vi "S2DS_ReadScript.vi"(7 "Data save info (in)":T1={"File path"=path "", "Header"="", "File name"="", "False channel"=[], "Channel names"=[], "Buffer size"=0, "Format"="%.6f"}, 10 "All channel parameters":T2 {"Scan parameters"."Y data taking" items=["in both direction", "in up direction only", "in down direction only"]; "Scan parameters"."X data taking" items=["in both direction", "in up direction only", "in down direction only"]}, 11 "Status":refnum<vi>) -> (0 "Full Status":string, 1 "update instruction":i32[](array[numeric])=[0, 1, 2, 3, 4], 2 "All channel parameters (out)":T2 {"Scan parameters"."Y data taking" items=["in both direction", "in up direction only", "in down direction only"]; "Scan parameters"."X data taking" items=["in both direction", "in up direction only", "in down direction only"]}, 3 "Script complete?":bool, 5 "Data save info (out)":T1={"File path"=path "", "Header"="", "File name"="", "False channel"=[], "Channel names"=[], "Buffer size"=0, "Format"="%.6f"})   [LabVIEW 2025]
uses:
  TYPE DEFS/S2DS_All Channel Parameters.ctl
  TYPE DEFS/S2DS_WC info.ctl
  TYPE DEFS/S2DS_Single WC info.ctl
  TYPE DEFS/S2DS_RC info.ctl
  TYPE DEFS/S2DS_Single RC info.ctl
  TYPE DEFS/S2DS_DAC info new.ctl
  TYPE DEFS/S2DS_Single DC info.ctl
  TYPE DEFS/S2DS_Array Inst Info.ctl
  TYPE DEFS/S2DS_Sweep Info.ctl
  TYPE DEFS/S2DS_Data saving info.ctl
  <vilib>/Utility/error.llb/Trim Whitespace One-Sided.vi
  <vilib>/Utility/config.llb/Read Key (Path).vi
  <vilib>/Utility/config.llb/Read Key (I32).vi
  <vilib>/Utility/config.llb/Write Key (Path).vi
  <vilib>/Utility/config.llb/Read Key (String).vi
  <vilib>/Utility/config.llb/Write Key (I32).vi
  <vilib>/Utility/config.llb/NI_LVConfig.lvlib
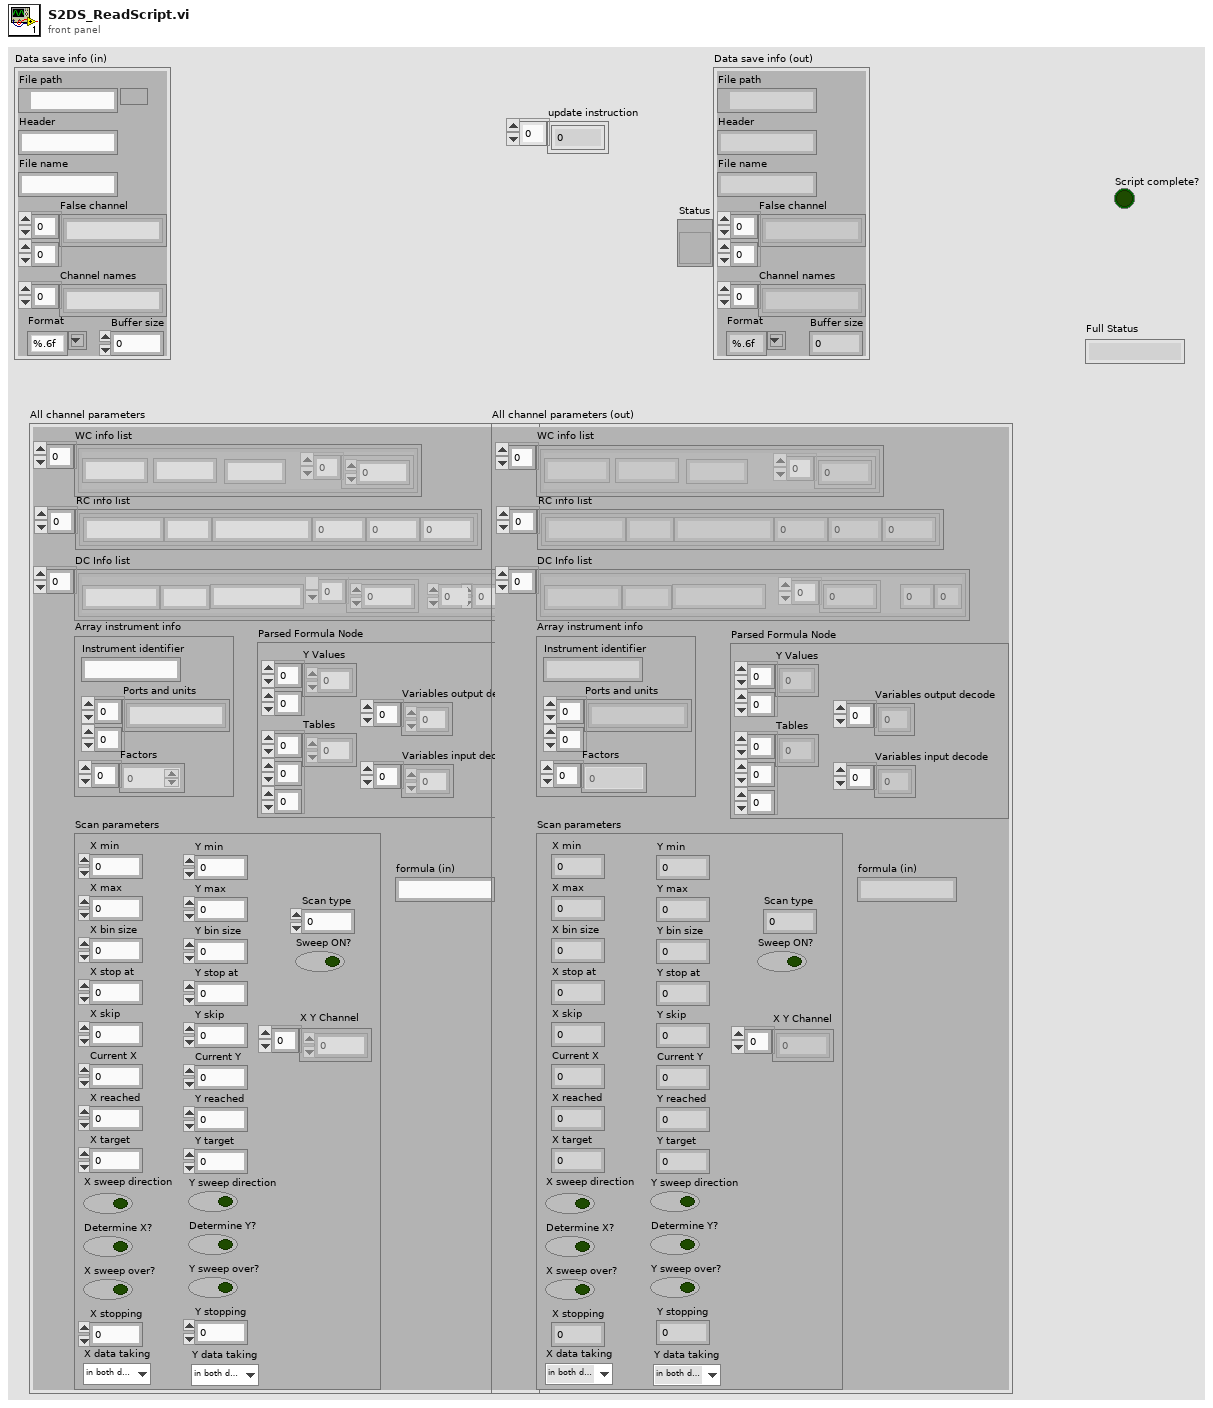
[diagram p1: front panel]
types:
  T1 = typedef "S2DS_Data saving info.ctl" = cluster{"File path":path, "Header":string, "File name":string, "False channel":string[][], "Channel names":string[], "Buffer size":i32, "Format":string}
  T2 = typedef "S2DS_All Channel Parameters.ctl" = cluster{"WC info list":T3, "RC info list":T5, "DC Info list":T7, "Array instrument info":T9, "Scan parameters":T10, "Parsed Formula Node":cluster{"Y Values":dbl[][], "Tables":i32[][][], "Variables input decode":i32[], "Variables output decode":i32[]}, "formula (in)":string}
  T3 = typedef "S2DS_WC info.ctl" = T4[]
  T4 = typedef "S2DS_Single WC info.ctl" = cluster{"Instrument identifier":string, "Write channel parameters":dbl[], "Name":string, "Unit":string}
  T5 = typedef "S2DS_RC info.ctl" = T6[]
  T6 = typedef "S2DS_Single RC info.ctl" = cluster{"Instrument identifier":string, "Factor":dbl, "Averaging":i32, "Wait (ms)":i32, "Unit":string, "Name":string}
  T7 = typedef "S2DS_DAC info new.ctl" = T8[]
  T8 = typedef "S2DS_Single DC info.ctl" = cluster{"Operation identifier":string, "DC parameters":dbl[], "U":i32, "V":i32, "Name":string, "Unit":string}
  T9 = typedef "S2DS_Array Inst Info.ctl" = cluster{"Instrument identifier":string, "Ports and units":string[][], "Factors":dbl[]}
  T10 = typedef "S2DS_Sweep Info.ctl" = cluster{"X min":ext, "X max":dbl, "Y min":dbl, "Y max":dbl, "X bin size":dbl, "Y bin size":dbl, "X stop at":dbl, "Y stop at":dbl, "X skip":u64, "Y skip":u64, "Current X":dbl, "Current Y":dbl, "X reached":i32, "Y reached":i32, "X target":dbl, "Y target":dbl, "Sweep ON?":bool, "X sweep direction":bool, "Y sweep direction":bool, "Determine X?":bool, "Determine Y?":bool, "X sweep over?":bool, "Y sweep over?":bool, "Scan type":i32, "X stopping":i32, "Y stopping":i32, "X Y Channel":u16[], "X data taking":u16, "Y data taking":u16}
  T11 = typedef "NI_LVConfig.lvlib/Config Data RefNum.ctl" = refnum<k1>
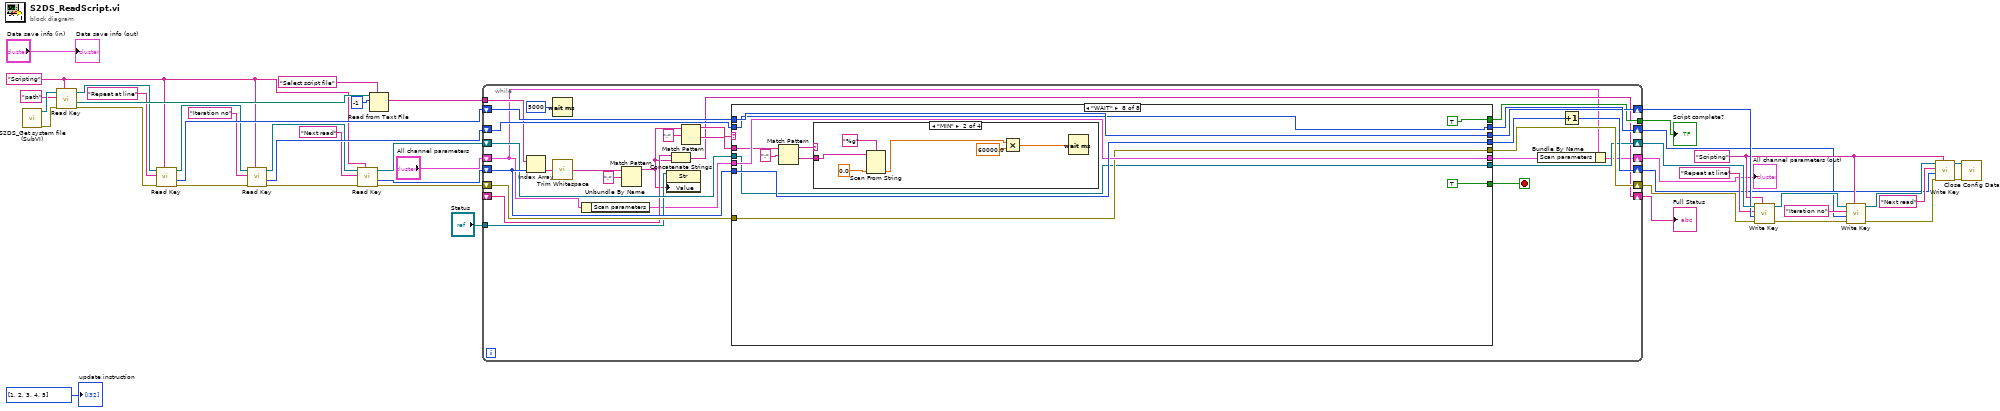
[diagram p0: block diagram]
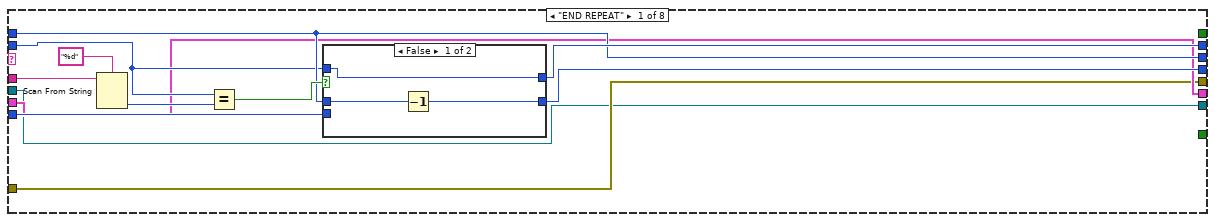
[diagram p2: hidden frame]
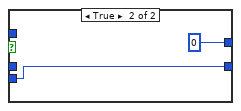
[diagram p3: hidden frame]
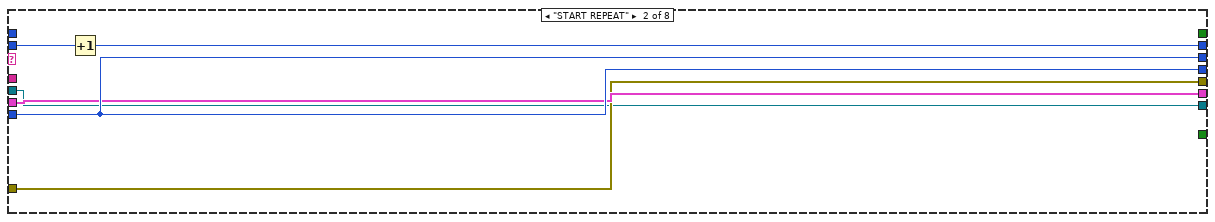
[diagram p4: hidden frame]
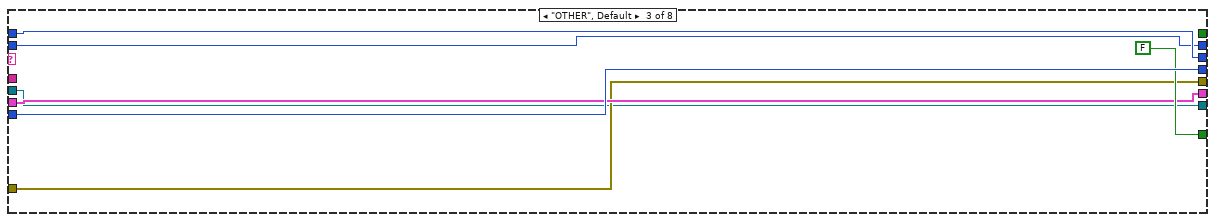
[diagram p5: hidden frame]
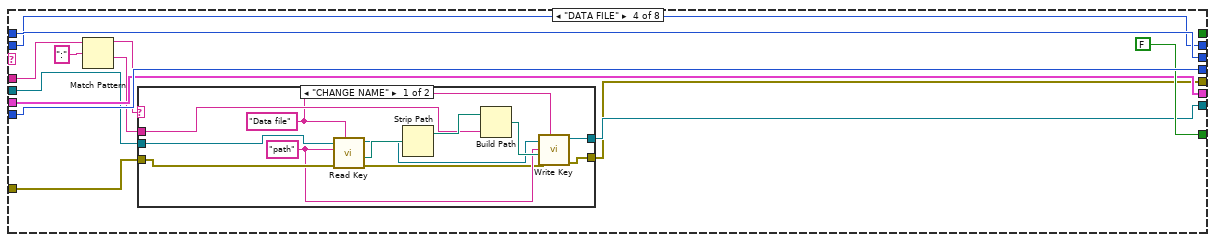
[diagram p6: hidden frame]
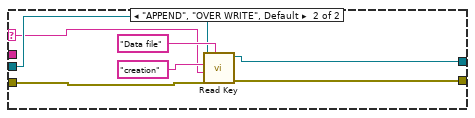
[diagram p7: hidden frame]
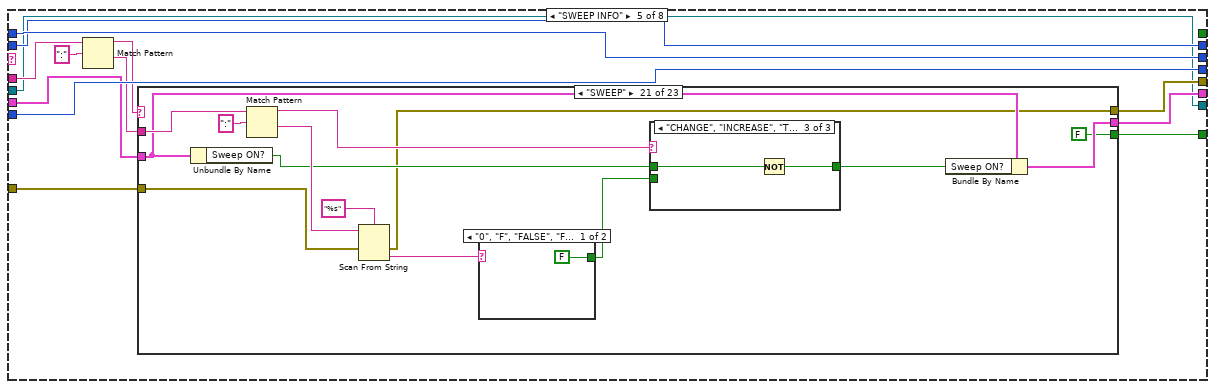
[diagram p8: hidden frame]
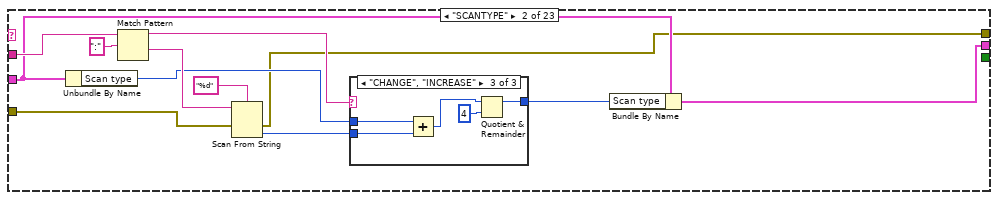
[diagram p10: hidden frame]
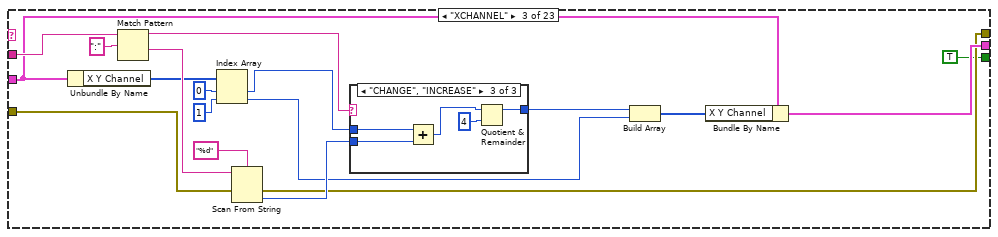
[diagram p13: hidden frame]
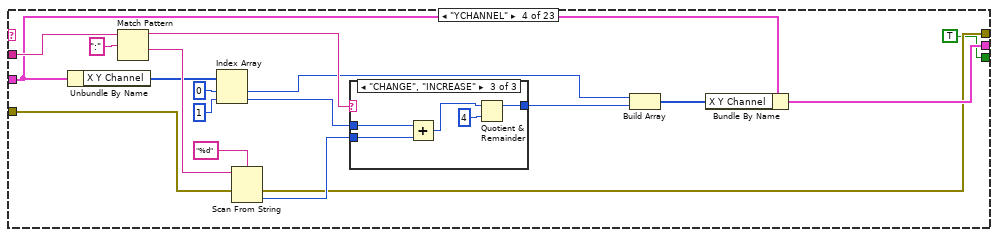
[diagram p16: hidden frame]
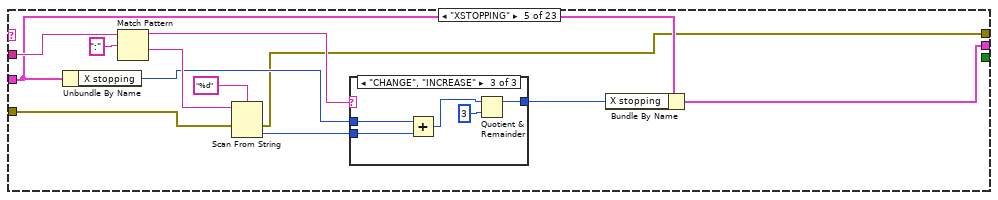
[diagram p19: hidden frame]
diagram:
  w12 = "Scripting" ("section")
  w27 = "Scripting" ("section")
  n1 = call "S2DS_Get system file (SubVI).vi"() -> ("error out"=w39:errorcluster, "Refnum out"=w40:T11)  [unwired: 10 in]
  n2 = call-poly <vilib>:"Read Key.vi"("section"=w27, "error in (no error)"=w39, "key"="path", "refnum"=w40) -> ("error out"=w35:errorcluster, "value"=w37:path, "refnum out"=w36:T11)  [unwired: 4 in, 1 out]
  n3 = call-poly <vilib>:"Read Key.vi"("section"=w27, "error in (no error)"=w35, "key"="Repeat at line", "refnum"=w36) -> ("error out"=w30:errorcluster, "value"=w33:i32, "refnum out"=w32:T11)  [unwired: 4 in, 1 out]
  n4 = call-poly <vilib>:"Read Key.vi"("section"=w27, "error in (no error)"=w30, "key"="Iteration no", "refnum"=w32) -> ("error out"=w25:errorcluster, "value"=w29:i32, "refnum out"=w28:T11)  [unwired: 4 in, 1 out]
  n5 = call-poly <vilib>:"Read Key.vi"("section"=w27, "error in (no error)"=w25, "key"="Next read", "refnum"=w28) -> ("error out"=w23:errorcluster, "value"=w24:i32, "refnum out"=w22:T11)  [unwired: 4 in, 1 out]
  n6 = Read from Text File(prompt (Open existing file)="Select script file" ("prompt"), file (use dialog)=w37, count=-1) -> (text=w42:string[])  [unwired: 1 in, 3 out]
  n7 = while {
    tunnel: w42 -> [w66]
    shift-right: [w69] -> w5
    shift-left: w29 -> [w70]
    shift-right: [w62] -> w6
    shift-left: w24 -> [w65]
    shift-right: [w68] -> w19
    shift-left: w33 -> [w67]
    tunnel: [w57] -> w41
    shift-right: [w45] -> w2
    shift-left: "All channel parameters" -> [w47]
    shift-right: [w55] -> w20
    shift-left: w23 -> [w56]
    shift-right: [w53] -> w21
    shift-left: w22 -> [w54]
    shift-right: [w51] -> w8
    shift-left: _ -> [w52]
    tunnel: "Status" -> [w50]
    stop <- w61 stop-if-true
    n8 = Index Array(array=w66, index=w65) -> (element=w64:string)
    n9 = Wait (ms)(milliseconds to wait=u32 5000) -> ()  [unwired: 1 out]
    n10 = call <vilib>:"Trim Whitespace.vi"("string"=w64) -> ("trimmed string"=w59:string)  [unwired: 1 in]
    n11 = Unbundle By Name(w47) -> ("Scan parameters"=w48:T10)
    n12 = Match Pattern(string=w59, regular expression=";") -> (before substring=w49:string)  [unwired: 1 in, 3 out]
    n13 = property on="Property Node" class="Str"(reference=w50, "Value"=w49) -> ()  [unwired: 1 in, 2 out]
    n14 = Concatenate Strings(w52, w49) -> (w51:string)
    n15 = Match Pattern(string=w49, regular expression=":") -> (before substring=w60:string, after substring=w71:string)  [unwired: 1 in, 2 out]
    n16 = case shown="\"WAIT\"" w60 {
      tunnel: w71 -> [w83 _ _ w110 w145 _ _ w571]
      tunnel: w70 -> [w77 w96 w101 w114 w146 w558 w566 w578]
      tunnel: [w79 w95 w101 w114 w146 w558 w566 w578] -> w69
      tunnel: [w78 w94 w102 w115 w147 w559 w567 w579] -> w68
      tunnel: w65 -> [w85 w94 w103 w116 w148 w560 w568 w580]
      tunnel: w67 -> [w78 _ w102 w115 w147 w559 w567 w579]
      tunnel: [w84 w94 w103 w116 w148 w560 w568 w580] -> w63
      tunnel: [_ _ FALSE FALSE w137 TRUE TRUE TRUE] -> w61
      tunnel: [_ _ _ _ _ _ TRUE TRUE] -> w57
      tunnel: w48 -> [w76 w93 w99 w112 w142 w556 w563 w575]
      tunnel: [w76 w93 w99 w112 w141 w556 w563 w575] -> w46
      tunnel: w56 -> [w75 w92 w98 w105 w140 w555 w562 w574]
      tunnel: [w75 w92 w98 w104 w139 w555 w562 w574] -> w55
      tunnel: w54 -> [w74 w91 w97 w108 w136 w554 w561 w573]
      tunnel: [w74 w91 w97 w106 w136 w554 w561 w573] -> w53
      frame "END REPEAT" {
        n17 = Scan From String(format string="%d", input string=w83) -> (output 1=w81:i32)  [unwired: 3 in, 3 out]
        n18 = Equal?(x=w77, y=w81) -> (x = y?=w80:bool)
        n19 = case shown="False" w80 {
          tunnel: w85 -> [_ w89]
          tunnel: [w86 w89] -> w84
          tunnel: w78 -> [w87 _]
          tunnel: [w88 0] -> w79
          tunnel: w77 -> [w88 _]
          frame False {
            n20 = Decrement(x=w87) -> (x-1=w86:i32)
          }
          frame True {
          }
        }
      }
      frame "START REPEAT" {
        n21 = Increment(x=w96) -> (x+1=w95:i32)
      }
      frame "OTHER", Default {
      }
      frame "DATA FILE" {
        n22 = Match Pattern(string=w110, regular expression=":") -> (before substring=w109:string, after substring=w107:string)  [unwired: 1 in, 2 out]
        n23 = case shown="\"CHANGE NAME\"" w109 {
          selector: w109 -> [_ w131]
          tunnel: w107 -> [w124 _]
          tunnel: w108 -> [w128 w133]
          tunnel: w105 -> [w127 w132]
          tunnel: [w118 w130] -> w106
          tunnel: [w117 w129] -> w104
          frame "CHANGE NAME" {
            w121 = "path" ("key")
            w122 = "Data file" ("section")
            n24 = call-poly <vilib>:"Read Key.vi"("section"=w122, "error in (no error)"=w127, "key"=w121, "refnum"=w128) -> ("error out"=w119:errorcluster, "value"=w126:path, "refnum out"=w120:T11)  [unwired: 4 in, 1 out]
            n25 = Strip Path(path=w126) -> (stripped path=w125:path)  [unwired: 1 out]
            n26 = Build Path(base path=w125, name or relative path=w124) -> (appended path=w123:path)
            n27 = call-poly <vilib>:"Write Key.vi"("section"=w122, "error in (no error)"=w119, "value"=w123, "key"=w121, "refnum"=w120) -> ("error out"=w117:errorcluster, "refnum out"=w118:T11)  [unwired: 4 in, 1 out]
          }
          frame "APPEND", "OVER WRITE", Default {
            n28 = call-poly <vilib>:"Read Key.vi"("section"="Data file", "error in (no error)"=w132, "default value"=w131, "key"="creation", "refnum"=w133) -> ("error out"=w129:errorcluster, "refnum out"=w130:T11)  [unwired: 3 in, 2 out]
          }
        }
      }
      frame "SWEEP INFO" {
        n29 = Match Pattern(string=w145, regular expression=":") -> (before substring=w143:string, after substring=w138:string)  [unwired: 1 in, 2 out]
        n30 = case shown="\"SWEEP\"" w143 {
          tunnel: w138 -> [_ w162 w187 w212 w231 w250 w269 w286 w303 w320 w337 w354 w371 w388 w405 w422 w439 w456 w473 w490 w509 w528 w547]
          tunnel: w142 -> [w150 w157 w182 w207 w226 w245 w264 w281 w298 w315 w332 w349 w366 w383 w400 w417 w434 w451 w468 w485 w504 w523 w542]
          tunnel: [w150 w156 w181 w206 w225 w244 w263 w280 w297 w314 w331 w348 w365 w382 w399 w416 w433 w450 w467 w484 w503 w522 w541] -> w141
          tunnel: w140 -> [w149 w152 w179 w204 w221 w240 w259 w276 w293 w310 w327 w344 w361 w378 w395 w412 w429 w446 w463 w480 w500 w519 w538]
          tunnel: [w149 w151 w178 w203 w220 w239 w258 w275 w292 w309 w326 w343 w360 w377 w394 w411 w428 w445 w462 w479 w499 w518 w537] -> w139
          tunnel: [_ _ TRUE TRUE _ _ _ _ _ _ _ _ _ _ _ _ _ _ _ _ FALSE _ _] -> w137
          frame "False", Default {
          }
          frame "SCANTYPE" {
            n31 = Unbundle By Name(w157) -> ("Scan type"=w154:i32)
            n32 = Match Pattern(string=w162, regular expression=":") -> (before substring=w161:string, after substring=w159:string)  [unwired: 1 in, 2 out]
            n33 = Scan From String(format string="%d", input string=w159, error in=w152) -> (error out=w151:errorcluster, output 1=w153:i32)  [unwired: 2 in, 2 out]
            n34 = case shown="\"CHANGE\", \"INCREASE\"" w161 {
              tunnel: [w163 w164 w165] -> w155
              tunnel: w154 -> [w163 _ w168]
              tunnel: w153 -> [_ w164 w169]
              frame "False", Default {
              }
              frame "SET" {
              }
              frame "CHANGE", "INCREASE" {
                n35 = Add(x=w168, y=w169) -> (x+y=w167:i32)
                n36 = Quotient & Remainder(x=w167, y=4) -> (x-y*floor(x/y)=w165:i32)  [unwired: 1 out]
              }
            }
            n37 = Bundle By Name(cluster=w157, "Scan type"=w155) -> (w156:T10)
          }
          frame "XCHANNEL" {
            n38 = Unbundle By Name(w182) -> ("X Y Channel"=w177:u16[])
            n39 = Match Pattern(string=w187, regular expression=":") -> (before substring=w186:string, after substring=w184:string)  [unwired: 1 in, 2 out]
            n40 = Index Array(array=w177, index #1=0 ("index"), index #2=1 ("index")) -> (element #1=w174:u16, element #2=w172:u16)
            n41 = Scan From String(format string="%d", input string=w184, error in=w179) -> (error out=w178:errorcluster, output 1=w180:i32)  [unwired: 2 in, 2 out]
            n42 = case shown="\"CHANGE\", \"INCREASE\"" w186 {
              tunnel: [w188 w189 w190] -> w173
              tunnel: w174 -> [w188 _ w193]
              tunnel: w180 -> [_ w189 w194]
              frame "False", Default {
              }
              frame "SET" {
              }
              frame "CHANGE", "INCREASE" {
                n43 = Add(x=w193, y=w194) -> (x+y=w192:i32)
                n44 = Quotient & Remainder(x=w192, y=4) -> (x-y*floor(x/y)=w190:i32)  [unwired: 1 out]
              }
            }
            n45 = Build Array(w173, w172) -> (w171:i32[])
            n46 = Bundle By Name(cluster=w182, "X Y Channel"=w171) -> (w181:T10)
          }
          frame "YCHANNEL" {
            n47 = Unbundle By Name(w207) -> ("X Y Channel"=w202:u16[])
            n48 = Match Pattern(string=w212, regular expression=":") -> (before substring=w211:string, after substring=w209:string)  [unwired: 1 in, 2 out]
            n49 = Index Array(array=w202, index #1=0 ("index"), index #2=1 ("index")) -> (element #1=w196:u16, element #2=w198:u16)
            n50 = Scan From String(format string="%d", input string=w209, error in=w204) -> (error out=w203:errorcluster, output 1=w205:i32)  [unwired: 2 in, 2 out]
            n51 = case shown="\"CHANGE\", \"INCREASE\"" w211 {
              tunnel: [w213 w214 w215] -> w197
              tunnel: w198 -> [w213 _ w218]
              tunnel: w205 -> [_ w214 w219]
              frame "False", Default {
              }
              frame "SET" {
              }
              frame "CHANGE", "INCREASE" {
                n52 = Add(x=w218, y=w219) -> (x+y=w217:i32)
                n53 = Quotient & Remainder(x=w217, y=4) -> (x-y*floor(x/y)=w215:i32)  [unwired: 1 out]
              }
            }
            n54 = Build Array(w196, w197) -> (w199:i32[])
            n55 = Bundle By Name(cluster=w207, "X Y Channel"=w199) -> (w206:T10)
          }
          frame "XSTOPPING" {
            n56 = Unbundle By Name(w226) -> ("X stopping"=w223:i32)
            n57 = Match Pattern(string=w231, regular expression=":") -> (before substring=w230:string, after substring=w228:string)  [unwired: 1 in, 2 out]
            n58 = Scan From String(format string="%d", input string=w228, error in=w221) -> (error out=w220:errorcluster, output 1=w222:i32)  [unwired: 2 in, 2 out]
            n59 = case shown="\"CHANGE\", \"INCREASE\"" w230 {
              tunnel: [w232 w233 w234] -> w224
              tunnel: w223 -> [w232 _ w237]
              tunnel: w222 -> [_ w233 w238]
              frame "False", Default {
              }
              frame "SET" {
              }
              frame "CHANGE", "INCREASE" {
                n60 = Add(x=w237, y=w238) -> (x+y=w236:i32)
                n61 = Quotient & Remainder(x=w236, y=3) -> (x-y*floor(x/y)=w234:i32)  [unwired: 1 out]
              }
            }
            n62 = Bundle By Name(cluster=w226, "X stopping"=w224) -> (w225:T10)
          }
          frame "YSTOPPING" {
            n63 = Unbundle By Name(w245) -> ("Y stopping"=w242:i32)
            n64 = Match Pattern(string=w250, regular expression=":") -> (before substring=w249:string, after substring=w247:string)  [unwired: 1 in, 2 out]
            n65 = Scan From String(format string="%d", input string=w247, error in=w240) -> (error out=w239:errorcluster, output 1=w241:i32)  [unwired: 2 in, 2 out]
            n66 = case shown="\"CHANGE\", \"INCREASE\"" w249 {
              tunnel: [w251 w252 w253] -> w243
              tunnel: w242 -> [w251 _ w256]
              tunnel: w241 -> [_ w252 w257]
              frame "False", Default {
              }
              frame "SET" {
              }
              frame "CHANGE", "INCREASE" {
                n67 = Add(x=w256, y=w257) -> (x+y=w255:i32)
                n68 = Quotient & Remainder(x=w255, y=3) -> (x-y*floor(x/y)=w253:i32)  [unwired: 1 out]
              }
            }
            n69 = Bundle By Name(cluster=w245, "Y stopping"=w243) -> (w244:T10)
          }
          frame "XMIN" {
            n70 = Unbundle By Name(w264) -> ("X min"=w261:ext)
            n71 = Match Pattern(string=w269, regular expression=":") -> (before substring=w268:string, after substring=w266:string)  [unwired: 1 in, 2 out]
            n72 = Scan From String(format string="%g", input string=w266, error in=w259) -> (error out=w258:errorcluster, output 1=w260:dbl)  [unwired: 2 in, 2 out]
            n73 = case shown="\"CHANGE\", \"INCREASE\"" w268 {
              tunnel: [w270 w271 w272] -> w262
              tunnel: w261 -> [w270 _ w273]
              tunnel: w260 -> [_ w271 w274]
              frame "False", Default {
              }
              frame "SET" {
              }
              frame "CHANGE", "INCREASE" {
                n74 = Add(x=w273, y=w274) -> (x+y=w272:ext)
              }
            }
            n75 = Bundle By Name(cluster=w264, "X min"=w262) -> (w263:T10)
          }
          frame "XMAX" {
            n76 = Unbundle By Name(w281) -> ("X max"=w278:dbl)
            n77 = Match Pattern(string=w286, regular expression=":") -> (before substring=w285:string, after substring=w283:string)  [unwired: 1 in, 2 out]
            n78 = Scan From String(format string="%g", input string=w283, error in=w276) -> (error out=w275:errorcluster, output 1=w277:dbl)  [unwired: 2 in, 2 out]
            n79 = case shown="\"CHANGE\", \"INCREASE\"" w285 {
              tunnel: [w287 w288 w289] -> w279
              tunnel: w278 -> [w287 _ w290]
              tunnel: w277 -> [_ w288 w291]
              frame "False", Default {
              }
              frame "SET" {
              }
              frame "CHANGE", "INCREASE" {
                n80 = Add(x=w290, y=w291) -> (x+y=w289:dbl)
              }
            }
            n81 = Bundle By Name(cluster=w281, "X max"=w279) -> (w280:T10)
          }
          frame "YMIN" {
            n82 = Unbundle By Name(w298) -> ("Y min"=w295:dbl)
            n83 = Match Pattern(string=w303, regular expression=":") -> (before substring=w302:string, after substring=w300:string)  [unwired: 1 in, 2 out]
            n84 = Scan From String(format string="%g", input string=w300, error in=w293) -> (error out=w292:errorcluster, output 1=w294:dbl)  [unwired: 2 in, 2 out]
            n85 = case shown="\"CHANGE\", \"INCREASE\"" w302 {
              tunnel: [w304 w305 w306] -> w296
              tunnel: w295 -> [w304 _ w307]
              tunnel: w294 -> [_ w305 w308]
              frame "False", Default {
              }
              frame "SET" {
              }
              frame "CHANGE", "INCREASE" {
                n86 = Add(x=w307, y=w308) -> (x+y=w306:dbl)
              }
            }
            n87 = Bundle By Name(cluster=w298, "Y min"=w296) -> (w297:T10)
          }
          frame "YMAX" {
            n88 = Unbundle By Name(w315) -> ("Y max"=w312:dbl)
            n89 = Match Pattern(string=w320, regular expression=":") -> (before substring=w319:string, after substring=w317:string)  [unwired: 1 in, 2 out]
            n90 = Scan From String(format string="%g", input string=w317, error in=w310) -> (error out=w309:errorcluster, output 1=w311:dbl)  [unwired: 2 in, 2 out]
            n91 = case shown="\"CHANGE\", \"INCREASE\"" w319 {
              tunnel: [w321 w322 w323] -> w313
              tunnel: w312 -> [w321 _ w324]
              tunnel: w311 -> [_ w322 w325]
              frame "False", Default {
              }
              frame "SET" {
              }
              frame "CHANGE", "INCREASE" {
                n92 = Add(x=w324, y=w325) -> (x+y=w323:dbl)
              }
            }
            n93 = Bundle By Name(cluster=w315, "Y max"=w313) -> (w314:T10)
          }
          frame "XBIN" {
            n94 = Unbundle By Name(w332) -> ("X bin size"=w329:dbl)
            n95 = Match Pattern(string=w337, regular expression=":") -> (before substring=w336:string, after substring=w334:string)  [unwired: 1 in, 2 out]
            n96 = Scan From String(format string="%g", input string=w334, error in=w327) -> (error out=w326:errorcluster, output 1=w328:dbl)  [unwired: 2 in, 2 out]
            n97 = case shown="\"CHANGE\", \"INCREASE\"" w336 {
              tunnel: [w338 w339 w340] -> w330
              tunnel: w329 -> [w338 _ w341]
              tunnel: w328 -> [_ w339 w342]
              frame "False", Default {
              }
              frame "SET" {
              }
              frame "CHANGE", "INCREASE" {
                n98 = Add(x=w341, y=w342) -> (x+y=w340:dbl)
              }
            }
            n99 = Bundle By Name(cluster=w332, "X bin size"=w330) -> (w331:T10)
          }
          frame "YBIN" {
            n100 = Unbundle By Name(w349) -> ("Y bin size"=w346:dbl)
            n101 = Match Pattern(string=w354, regular expression=":") -> (before substring=w353:string, after substring=w351:string)  [unwired: 1 in, 2 out]
            n102 = Scan From String(format string="%g", input string=w351, error in=w344) -> (error out=w343:errorcluster, output 1=w345:dbl)  [unwired: 2 in, 2 out]
            n103 = case shown="\"CHANGE\", \"INCREASE\"" w353 {
              tunnel: [w355 w356 w357] -> w347
              tunnel: w346 -> [w355 _ w358]
              tunnel: w345 -> [_ w356 w359]
              frame "False", Default {
              }
              frame "SET" {
              }
              frame "CHANGE", "INCREASE" {
                n104 = Add(x=w358, y=w359) -> (x+y=w357:dbl)
              }
            }
            n105 = Bundle By Name(cluster=w349, "Y bin size"=w347) -> (w348:T10)
          }
          frame "XSTOPPAGE" {
            n106 = Unbundle By Name(w366) -> ("X stop at"=w363:dbl)
            n107 = Match Pattern(string=w371, regular expression=":") -> (before substring=w370:string, after substring=w368:string)  [unwired: 1 in, 2 out]
            n108 = Scan From String(format string="%g", input string=w368, error in=w361) -> (error out=w360:errorcluster, output 1=w362:dbl)  [unwired: 2 in, 2 out]
            n109 = case shown="\"CHANGE\", \"INCREASE\"" w370 {
              tunnel: [w372 w373 w374] -> w364
              tunnel: w363 -> [w372 _ w375]
              tunnel: w362 -> [_ w373 w376]
              frame "False", Default {
              }
              frame "SET" {
              }
              frame "CHANGE", "INCREASE" {
                n110 = Add(x=w375, y=w376) -> (x+y=w374:dbl)
              }
            }
            n111 = Bundle By Name(cluster=w366, "X stop at"=w364) -> (w365:T10)
          }
          frame "YSTOPPAGE" {
            n112 = Unbundle By Name(w383) -> ("Y stop at"=w380:dbl)
            n113 = Match Pattern(string=w388, regular expression=":") -> (before substring=w387:string, after substring=w385:string)  [unwired: 1 in, 2 out]
            n114 = Scan From String(format string="%g", input string=w385, error in=w378) -> (error out=w377:errorcluster, output 1=w379:dbl)  [unwired: 2 in, 2 out]
            n115 = case shown="\"CHANGE\", \"INCREASE\"" w387 {
              tunnel: [w389 w390 w391] -> w381
              tunnel: w380 -> [w389 _ w392]
              tunnel: w379 -> [_ w390 w393]
              frame "False", Default {
              }
              frame "SET" {
              }
              frame "CHANGE", "INCREASE" {
                n116 = Add(x=w392, y=w393) -> (x+y=w391:dbl)
              }
            }
            n117 = Bundle By Name(cluster=w383, "Y stop at"=w381) -> (w382:T10)
          }
          frame "XSKIP" {
            n118 = Unbundle By Name(w400) -> ("X skip"=w397:u64)
            n119 = Match Pattern(string=w405, regular expression=":") -> (before substring=w404:string, after substring=w402:string)  [unwired: 1 in, 2 out]
            n120 = Scan From String(format string="%g", input string=w402, error in=w395) -> (error out=w394:errorcluster, output 1=w396:dbl)  [unwired: 2 in, 2 out]
            n121 = case shown="\"CHANGE\", \"INCREASE\"" w404 {
              tunnel: [w406 w407 w408] -> w398
              tunnel: w397 -> [w406 _ w409]
              tunnel: w396 -> [_ w407 w410]
              frame "False", Default {
              }
              frame "SET" {
              }
              frame "CHANGE", "INCREASE" {
                n122 = Add(x=w409, y=w410) -> (x+y=w408:dbl)
              }
            }
            n123 = Bundle By Name(cluster=w400, "X skip"=w398) -> (w399:T10)
          }
          frame "YSKIP" {
            n124 = Unbundle By Name(w417) -> ("Y skip"=w414:u64)
            n125 = Match Pattern(string=w422, regular expression=":") -> (before substring=w421:string, after substring=w419:string)  [unwired: 1 in, 2 out]
            n126 = Scan From String(format string="%g", input string=w419, error in=w412) -> (error out=w411:errorcluster, output 1=w413:dbl)  [unwired: 2 in, 2 out]
            n127 = case shown="\"CHANGE\", \"INCREASE\"" w421 {
              tunnel: [w423 w424 w425] -> w415
              tunnel: w414 -> [w423 _ w426]
              tunnel: w413 -> [_ w424 w427]
              frame "False", Default {
              }
              frame "SET" {
              }
              frame "CHANGE", "INCREASE" {
                n128 = Add(x=w426, y=w427) -> (x+y=w425:dbl)
              }
            }
            n129 = Bundle By Name(cluster=w417, "Y skip"=w415) -> (w416:T10)
          }
          frame "XPRESENT" {
            n130 = Unbundle By Name(w434) -> ("Current X"=w431:dbl)
            n131 = Match Pattern(string=w439, regular expression=":") -> (before substring=w438:string, after substring=w436:string)  [unwired: 1 in, 2 out]
            n132 = Scan From String(format string="%g", input string=w436, error in=w429) -> (error out=w428:errorcluster, output 1=w430:dbl)  [unwired: 2 in, 2 out]
            n133 = case shown="\"CHANGE\", \"INCREASE\"" w438 {
              tunnel: [w440 w441 w442] -> w432
              tunnel: w431 -> [w440 _ w443]
              tunnel: w430 -> [_ w441 w444]
              frame "False", Default {
              }
              frame "SET" {
              }
              frame "CHANGE", "INCREASE" {
                n134 = Add(x=w443, y=w444) -> (x+y=w442:dbl)
              }
            }
            n135 = Bundle By Name(cluster=w434, "Current X"=w432) -> (w433:T10)
          }
          frame "YPRESENT" {
            n136 = Unbundle By Name(w451) -> ("Current Y"=w448:dbl)
            n137 = Match Pattern(string=w456, regular expression=":") -> (before substring=w455:string, after substring=w453:string)  [unwired: 1 in, 2 out]
            n138 = Scan From String(format string="%g", input string=w453, error in=w446) -> (error out=w445:errorcluster, output 1=w447:dbl)  [unwired: 2 in, 2 out]
            n139 = case shown="\"CHANGE\", \"INCREASE\"" w455 {
              tunnel: [w457 w458 w459] -> w449
              tunnel: w448 -> [w457 _ w460]
              tunnel: w447 -> [_ w458 w461]
              frame "False", Default {
              }
              frame "SET" {
              }
              frame "CHANGE", "INCREASE" {
                n140 = Add(x=w460, y=w461) -> (x+y=w459:dbl)
              }
            }
            n141 = Bundle By Name(cluster=w451, "Current Y"=w449) -> (w450:T10)
          }
          frame "XTARGET" {
            n142 = Unbundle By Name(w468) -> ("X target"=w465:dbl)
            n143 = Match Pattern(string=w473, regular expression=":") -> (before substring=w472:string, after substring=w470:string)  [unwired: 1 in, 2 out]
            n144 = Scan From String(format string="%g", input string=w470, error in=w463) -> (error out=w462:errorcluster, output 1=w464:dbl)  [unwired: 2 in, 2 out]
            n145 = case shown="\"CHANGE\", \"INCREASE\"" w472 {
              tunnel: [w474 w475 w476] -> w466
              tunnel: w465 -> [w474 _ w477]
              tunnel: w464 -> [_ w475 w478]
              frame "False", Default {
              }
              frame "SET" {
              }
              frame "CHANGE", "INCREASE" {
                n146 = Add(x=w477, y=w478) -> (x+y=w476:dbl)
              }
            }
            n147 = Bundle By Name(cluster=w468, "X target"=w466) -> (w467:T10)
          }
          frame "YTARGET" {
            n148 = Unbundle By Name(w485) -> ("Y target"=w482:dbl)
            n149 = Match Pattern(string=w490, regular expression=":") -> (before substring=w489:string, after substring=w487:string)  [unwired: 1 in, 2 out]
            n150 = Scan From String(format string="%g", input string=w487, error in=w480) -> (error out=w479:errorcluster, output 1=w481:dbl)  [unwired: 2 in, 2 out]
            n151 = case shown="\"CHANGE\", \"INCREASE\"" w489 {
              tunnel: [w491 w492 w493] -> w483
              tunnel: w482 -> [w491 _ w494]
              tunnel: w481 -> [_ w492 w495]
              frame "False", Default {
              }
              frame "SET" {
              }
              frame "CHANGE", "INCREASE" {
                n152 = Add(x=w494, y=w495) -> (x+y=w493:dbl)
              }
            }
            n153 = Bundle By Name(cluster=w485, "Y target"=w483) -> (w484:T10)
          }
          frame "SWEEP" {
            n154 = Unbundle By Name(w504) -> ("Sweep ON?"=w501:bool)
            n155 = Match Pattern(string=w509, regular expression=":") -> (before substring=w508:string, after substring=w506:string)  [unwired: 1 in, 2 out]
            n156 = Scan From String(format string="%s", input string=w506, error in=w500) -> (error out=w499:errorcluster, output 1=w498:string)  [unwired: 2 in, 2 out]
            n157 = case shown="\"0\", \"F\", \"FALSE\", \"False\", Default" w498 {
              tunnel: [FALSE TRUE] -> w497
              frame "0", "F", "FALSE", "False", Default {
              }
              frame "1", "T", "TRUE", "True" {
              }
            }
            n158 = case shown="\"CHANGE\", \"INCREASE\", \"TOGGLE\"" w508 {
              tunnel: [w512 w513 w514] -> w502
              tunnel: w501 -> [w512 _ w515]
              tunnel: w497 -> [_ w513 _]
              frame "False", Default {
              }
              frame "SET" {
              }
              frame "CHANGE", "INCREASE", "TOGGLE" {
                n159 = Not(x=w515) -> (.not. x?=w514:bool)
              }
            }
            n160 = Bundle By Name(cluster=w504, "Sweep ON?"=w502) -> (w503:T10)
          }
          frame "XDIRECTION" {
            n161 = Unbundle By Name(w523) -> ("X sweep direction"=w520:bool)
            n162 = Match Pattern(string=w528, regular expression=":") -> (before substring=w527:string, after substring=w525:string)  [unwired: 1 in, 2 out]
            n163 = Scan From String(format string="%s", input string=w525, error in=w519) -> (error out=w518:errorcluster, output 1=w517:string)  [unwired: 2 in, 2 out]
            n164 = case shown="\"0\", \"F\", \"FALSE\", \"False\", Default" w517 {
              tunnel: [FALSE TRUE] -> w516
              frame "0", "F", "FALSE", "False", Default {
              }
              frame "1", "T", "TRUE", "True" {
              }
            }
            n165 = case shown="\"CHANGE\", \"INCREASE\", \"TOGGLE\"" w527 {
              tunnel: [w531 w532 w533] -> w521
              tunnel: w520 -> [w531 _ w534]
              tunnel: w516 -> [_ w532 _]
              frame "False", Default {
              }
              frame "SET" {
              }
              frame "CHANGE", "INCREASE", "TOGGLE" {
                n166 = Not(x=w534) -> (.not. x?=w533:bool)
              }
            }
            n167 = Bundle By Name(cluster=w523, "X sweep direction"=w521) -> (w522:T10)
          }
          frame "YDIRECTION" {
            n168 = Unbundle By Name(w542) -> ("Y sweep direction"=w539:bool)
            n169 = Match Pattern(string=w547, regular expression=":") -> (before substring=w546:string, after substring=w544:string)  [unwired: 1 in, 2 out]
            n170 = Scan From String(format string="%s", input string=w544, error in=w538) -> (error out=w537:errorcluster, output 1=w536:string)  [unwired: 2 in, 2 out]
            n171 = case shown="\"0\", \"F\", \"FALSE\", \"False\", Default" w536 {
              tunnel: [FALSE TRUE] -> w535
              frame "0", "F", "FALSE", "False", Default {
              }
              frame "1", "T", "TRUE", "True" {
              }
            }
            n172 = case shown="\"CHANGE\", \"INCREASE\", \"TOGGLE\"" w546 {
              tunnel: [w550 w551 w552] -> w540
              tunnel: w539 -> [w550 _ w553]
              tunnel: w535 -> [_ w551 _]
              frame "False", Default {
              }
              frame "SET" {
              }
              frame "CHANGE", "INCREASE", "TOGGLE" {
                n173 = Not(x=w553) -> (.not. x?=w552:bool)
              }
            }
            n174 = Bundle By Name(cluster=w542, "Y sweep direction"=w540) -> (w541:T10)
          }
        }
      }
      frame "EXIT" {
      }
      frame "END SCRIPT" {
      }
      frame "WAIT" {
        n175 = Match Pattern(string=w571, regular expression=":") -> (before substring=w570:string, after substring=w569:string)  [unwired: 1 in, 2 out]
        n176 = case shown="\"MIN\"" w570 {
          tunnel: w569 -> [_ w586 w592 w598]
          frame "False", Default {
          }
          frame "MIN" {
            n177 = Scan From String(format string="%g", input string=w586, default 1=0.0 ("default value 1")) -> (output 1=w583:dbl)  [unwired: 2 in, 3 out]
            n178 = Multiply(x=w583, y=60000.0) -> (x*y=w581:dbl)
            n179 = Wait (ms)(milliseconds to wait=w581) -> ()  [unwired: 1 out]
          }
          frame "H", "HH", "HOUR" {
            n180 = Scan From String(format string="%g", input string=w592, default 1=0.0 ("default value 1")) -> (output 1=w589:dbl)  [unwired: 2 in, 3 out]
            n181 = Multiply(x=w589, y=3600000.0) -> (x*y=w587:dbl)
            n182 = Wait (ms)(milliseconds to wait=w587) -> ()  [unwired: 1 out]
          }
          frame "SEC", "SECOND" {
            n183 = Scan From String(format string="%g", input string=w598, default 1=0.0 ("default value 1")) -> (output 1=w595:dbl)  [unwired: 2 in, 3 out]
            n184 = Multiply(x=w595, y=1000.0) -> (x*y=w593:dbl)
            n185 = Wait (ms)(milliseconds to wait=w593) -> ()  [unwired: 1 out]
          }
        }
      }
    }
    n186 = Bundle By Name(cluster=w47, "Scan parameters"=w46) -> (w45:T2)
    n187 = Increment(x=w63) -> (x+1=w62:i32)
  }
  "Script complete?" <- w41
  "Full Status" <- w8
  "All channel parameters (out)" <- w2
  n188 = call-poly <vilib>:"Write Key.vi"("section"=w12, "error in (no error)"=w20, "value"=w19, "key"="Repeat at line", "refnum"=w21) -> ("error out"=w16:errorcluster, "refnum out"=w17:T11)  [unwired: 4 in, 1 out]
  n189 = call-poly <vilib>:"Write Key.vi"("section"=w12, "error in (no error)"=w16, "value"=w5, "key"="Iteration no", "refnum"=w17) -> ("error out"=w13:errorcluster, "refnum out"=w14:T11)  [unwired: 4 in, 1 out]
  n190 = call-poly <vilib>:"Write Key.vi"("section"=w12, "error in (no error)"=w13, "value"=w6, "key"="Next read", "refnum"=w14) -> ("error out"=w9:errorcluster, "refnum out"=w10:T11)  [unwired: 4 in, 1 out]
  n191 = call <vilib>:"Close Config Data.vi"("error in (no error)"=w9, "refnum"=w10) -> ()  [unwired: 8 in, 2 out]
  "update instruction" <- i32[] [1, 2, 3, 4, 5]
  "Data save info (out)" <- "Data save info (in)"
